vi "SSH Execute Command.vi"(8 "Error In":errorcluster, 10 "Command":string, 11 "SSH Session":refnum<k24>) -> (0 "Error Out":errorcluster, 2 "Std Out":string, 3 "SSH Session":refnum<k24>)   [LabVIEW 2014, in "LMH-LINX.lvlib"]
uses:
  <vilib>/MakerHub/LINX/LMH-LINX.lvlib
  C:/Program Files (x86)/National Instruments/LabVIEW 2014/vi.lib/MakerHub/LINX/Resources/Renci.SshNet.dll
  Resources/Renci.SshNet.dll
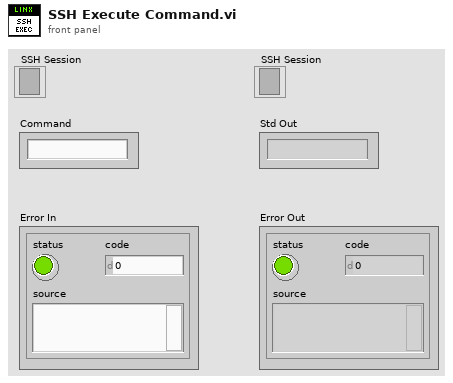
[diagram p1: front panel]
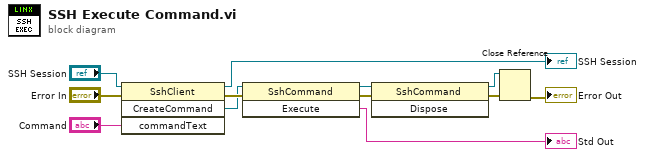
[diagram p0: block diagram]
diagram:
  n1 = invoke class="SshClient" method="CreateCommand"(reference="SSH Session", error in="Error In", "commandText"="Command") -> (reference out=→"SSH Session":refnum<k24>, error out=w12:errorcluster, "CreateCommand"=w5:refnum<k24>)  [unwired: 1 in, 1 out]
  n2 = invoke class="SshCommand" method="Execute"(reference=w5, error in=w12) -> (reference out=w11:refnum<k24>, error out=w10:errorcluster, "Execute"=→"Std Out":string)  [unwired: 1 in]
  n3 = invoke class="SshCommand" method="Dispose"(reference=w11, error in=w10) -> (reference out=w1:refnum<k24>, error out=w3:errorcluster)  [unwired: 1 in, 1 out]
  n4 = Close Reference(reference=w1, error in (no error)=w3) -> (error out=→"Error Out":errorcluster)
